vi "custom_2_stimulus_advanced.vi"(2 "Input Array":dbl[](array[numeric]), 3 "Cluster":T1) -> (0 "Timing array changed?":bool, 1 "Output Array":dbl[](array[numeric]))   [LabVIEW 2010]
panel:
  in  "Custom 2 Stimulul Duration(ms)":i32[][](array[numeric]) min=4 max=65535
  in  "Fraction of time between is active":dbl[][](array[numeric]) min=2.7272728356448087e-05
  in  "stop":bool
  in  "OK Button":bool
  in  "Custom 2 Stimulus Timing Array":dbl[](array[numeric])
  # "Duty Cycle"
  # "Switch time (ms)"
  # "Custom 2 Stimulus Timing Array (ms)"
  # "Trigger signal duration (ms)"
  # "Switch time (ms)"
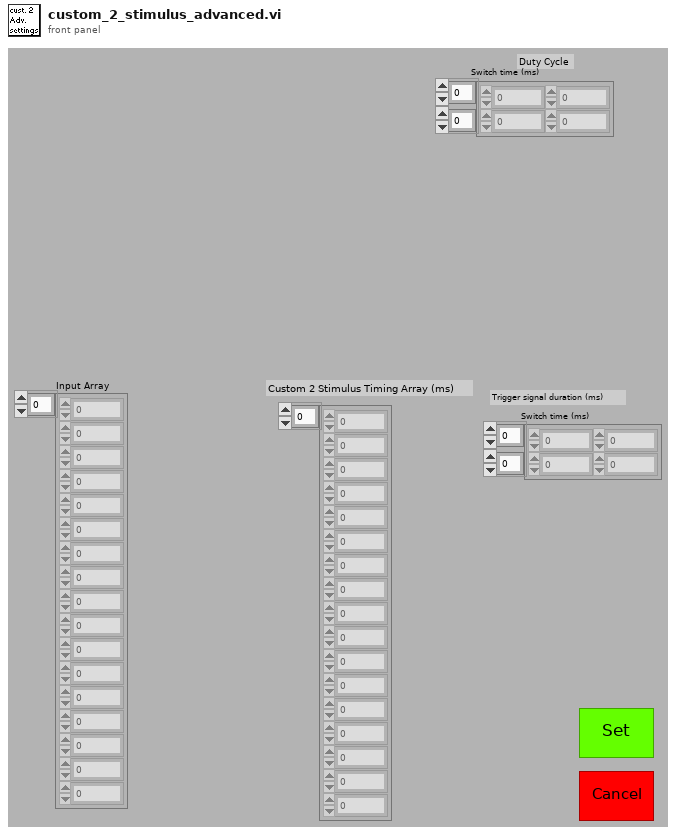
[diagram p1: front panel]
types:
  T1 = cluster{"custom 2 fraction of time between is active":refnum<vi>, "time between custom 2 onset":refnum<vi>}
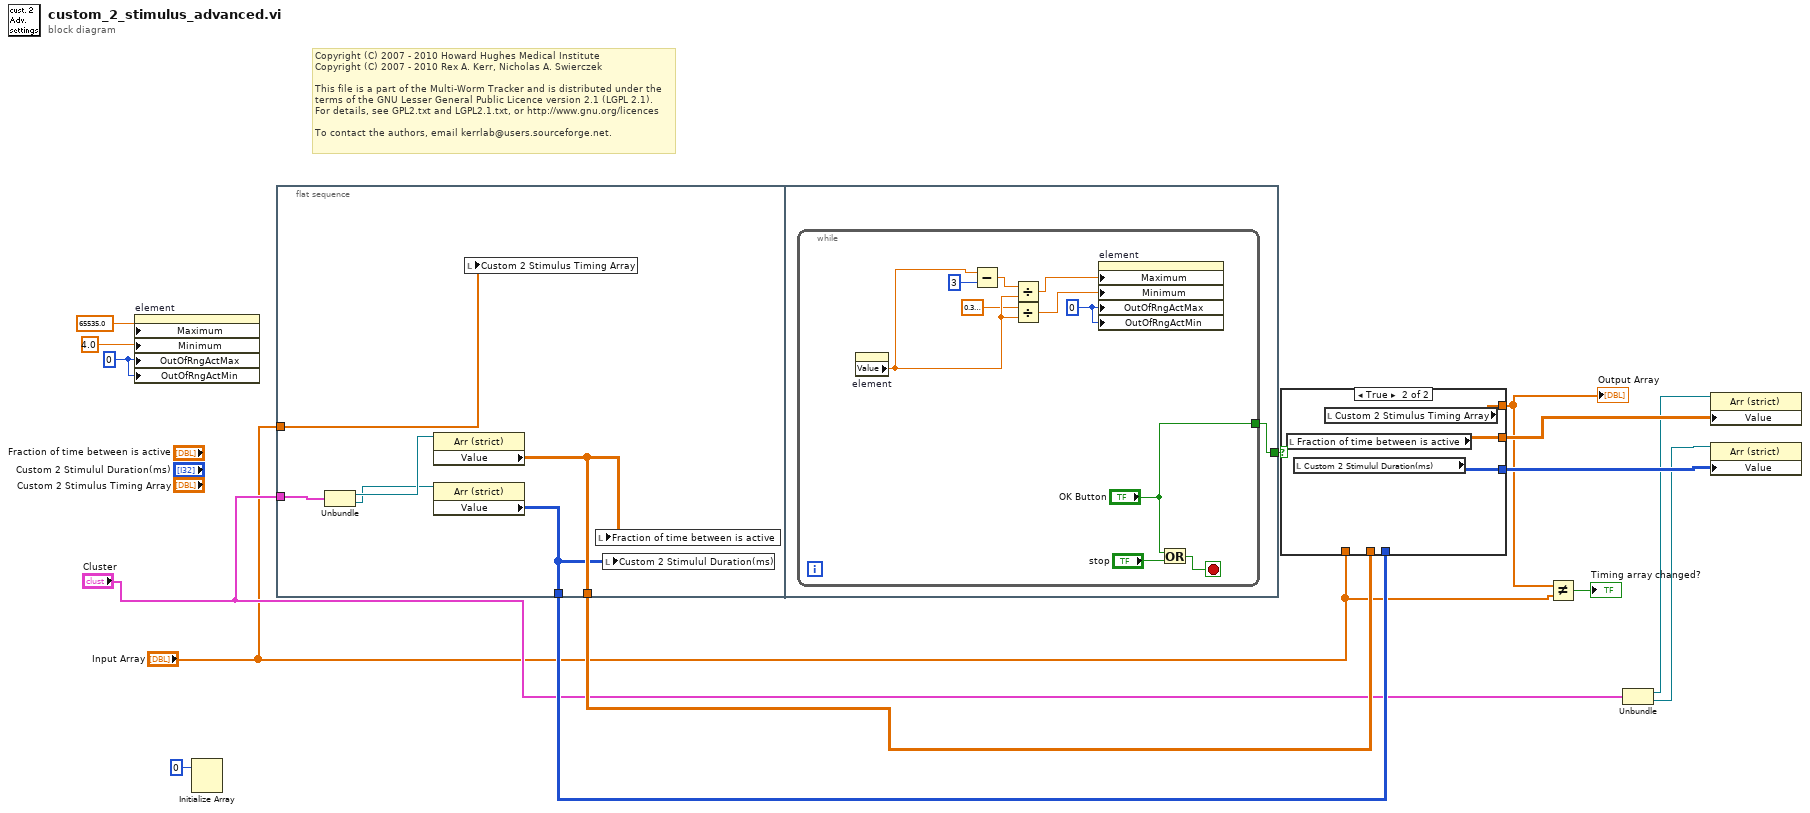
[diagram p0: block diagram]
diagram:
  w8 = u8 0 ("Response to Value Outside Limits:Maximum")
  # "Copyright (C) 2007 - 2010 Howard Hughes Medical Institute\nCopyright (C) 2007 - 2010 Rex A. Kerr, Nicholas A. Swierczek\n \nThis file is a part of the Multi-Worm Tracker and is distributed under the\nterms of the GNU Lesser General Public Licence version 2.1 (LGPL 2.1).\nFor details, see GPL2.txt and LGPL2.1.txt, or http://www.gnu.org/licences\n \nTo contact the authors, email kerrlab@users.sourceforge.net."
  n1 = property on="element" class="DigNum (strict)"("Maximum"=65535.0 ("x"), "Minimum"=4.0 ("Data Entry Limits:Minimum"), "OutOfRngActMax"=w8, "OutOfRngActMin"=w8) -> ()  [unwired: 2 in, 2 out]
  n2 = Initialize Array(0 ("element")) -> ()  [unwired: 2 in, 1 out]
  n3 = flat-sequence {
    tunnel: "Input Array" -> [w21]
    tunnel: "Cluster" -> [w20]
    tunnel: [w19] -> w7
    tunnel: [w18] -> w6
    tunnel: [w22] -> w15
    frame #0 {
      n4 = Unbundle(w20) -> ("custom 2 fraction of time between is active"=w17:refnum<vi>, "time between custom 2 onset"=w16:refnum<vi>)
      n5 = property class="Arr (strict)"(reference=w17) -> ("Value"=w19:sgl[][])  [unwired: 1 in, 2 out]
      n6 = property class="Arr (strict)"(reference=w16) -> ("Value"=w18:i32[][])  [unwired: 1 in, 2 out]
      n7 = local write "Custom 2 Stimulus Timing Array"(w21) -> ()
      n8 = local write "Fraction of time between is active"(w19) -> ()
      n9 = local write "Custom 2 Stimulul Duration(ms)"(w18) -> ()
    }
    frame #1 {
      n10 = while {
        tunnel: ["OK Button"] -> w22
        stop <- w32 stop-if-true
        w29 = u8 0 ("Response to Value Outside Limits:Maximum")
        n11 = property on="element" class="DigNum (strict)"() -> ("Value"=w28:dbl)  [unwired: 2 in, 2 out]
        n12 = Subtract(x=w28, y=3) -> (x-y=w26:dbl)
        n13 = Divide(x=w26, y=w28) -> (x/y=w27:dbl)
        n14 = Divide(x=sgl 0.3, y=w28) -> (x/y=w23:dbl)
        n15 = property on="element" class="DigNum (strict)"("Maximum"=w27, "Minimum"=w23, "OutOfRngActMax"=w29, "OutOfRngActMin"=w29) -> ()  [unwired: 2 in, 2 out]
        n16 = Or(x="OK Button", y="stop") -> (x .or. y?=w32:bool)
      }
    }
  }
  n17 = case shown="True" w15 {
    tunnel: "Input Array" -> [w35 _]
    tunnel: [w35 w38] -> w3
    tunnel: [w34 w37] -> w14
    tunnel: [w33 w36] -> w13
    tunnel: w7 -> [w34 _]
    tunnel: w6 -> [w33 _]
    frame False {
    }
    frame True {
      n18 = local read "Fraction of time between is active"() -> (w37:dbl[][])
      n19 = local read "Custom 2 Stimulul Duration(ms)"() -> (w36:i32[][])
      n20 = local read "Custom 2 Stimulus Timing Array"() -> (w38:dbl[])
    }
  }
  "Output Array" <- w3
  n21 = Not Equal?(x=w3, y="Input Array") -> (x != y?=→"Timing array changed?":bool)
  n22 = Unbundle("Cluster") -> ("custom 2 fraction of time between is active"=w12:refnum<vi>, "time between custom 2 onset"=w11:refnum<vi>)
  n23 = property class="Arr (strict)"(reference=w12, "Value"=w14) -> ()  [unwired: 1 in, 2 out]
  n24 = property class="Arr (strict)"(reference=w11, "Value"=w13) -> ()  [unwired: 1 in, 2 out]
